vi "SMC_GetLimit.vi"(8 "error in (no error)":errorcluster) -> (0 "error out":errorcluster, 2 "MaxValues":dbl[](array[numeric]) format="%.6f", 3 "MinValues":dbl[](array[numeric]) format="%.6f")   [LabVIEW 2015]
uses:
  SMC_SubVIs.llb/SMC_ManagerMode.ctl
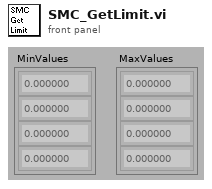
[diagram p1: front panel]
types:
  T1 = typedef "SMC_ManagerMode.ctl" = enum16{"Init", "Get", "SetPosition", "SetStatus", "SetMoving", "SetControllerNr"}
  T2 = typedef "SMC Paras.ctl" = cluster{"VENUS Language":T3, "Number of Axis":u8, "Controller Nr":u8, "Simulation":bool}
  T3 = typedef "VENUSNr.ctl" = enum16{"VENUS 2", "VENUS 1"}
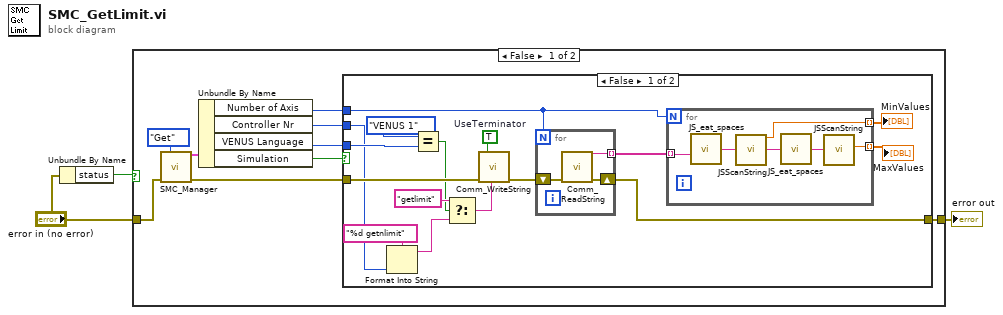
[diagram p0: block diagram]
diagram:
  n1 = Unbundle By Name("error in (no error)") -> ("status"=w3:bool)
  n2 = case shown="False" w3 {
    tunnel: "error in (no error)" -> [w11 w39]
    tunnel: [w9 w39] -> w1
    frame False {
      n3 = call "SMC_Manager.vi"("Mode"=SMC_ManagerMode."Get", "error in (no error)"=w11) -> ("SMC Parameter Out"=w8:T2, "error out"=w10:errorcluster)  [unwired: 9 in, 3 out]
      n4 = Unbundle By Name(w8) -> ("Number of Axis"=w5:u8, "Controller Nr"=w6:u8, "VENUS Language"=w7:T3, "Simulation"=w4:bool)
      n5 = case shown="False" w4 {
        tunnel: w10 -> [w25 w38]
        tunnel: [w23 w38] -> w9
        tunnel: w7 -> [w22 _]
        tunnel: w6 -> [w15 _]
        tunnel: w5 -> [w14 _]
        frame False {
          w13 = TRUE  # UseTerminator
          n6 = Format Into String(format string="%d getnlimit" ("Format String"), w15) -> (resulting string=w16:string)  [unwired: 2 in, 1 out]
          n7 = Equal?(x=enum16{"VENUS 2", "VENUS 1"}."VENUS 1", y=w22) -> (x = y?=w18:bool)
          n8 = Select(t="getlimit" ("Substring"), s=w18, f=w16) -> (s? t:f=w20:string)
          n9 = call "Comm_WriteString.vi"("string to write"=w20, "error in (no error)"=w25, "UseTerminator"=w13) -> ("error out"=w24:errorcluster)  [unwired: 8 in]
          n10 = for {
            N: w14 -> [_]
            shift-right: [w35] -> w23
            shift-left: w24 -> [w36]
            tunnel: [w37] -> w28 mode=indexing
            n11 = call "Comm_ReadString.vi"("error in (no error)"=w36) -> ("error out"=w35:errorcluster, "Answer"=w37:string)  [unwired: 9 in]
          }
          n12 = for {
            N: w14 -> [_]
            tunnel: [w31] -> w27 mode=indexing
            tunnel: w28 -> [w34] mode=indexing
            tunnel: [w30] -> w26 mode=indexing
            n13 = call "JS_eat_spaces.vi"("String In"=w34) -> ("String Out"=w33:string)
            n14 = call "JSScanString.vi"("String"=w33) -> ("result"=w31:dbl, "String Out"=w32:string)  [unwired: 9 in]
            n15 = call "JS_eat_spaces.vi"("String In"=w32) -> ("String Out"=w29:string)
            n16 = call "JSScanString.vi"("String"=w29) -> ("result"=w30:dbl)  [unwired: 9 in, 1 out]
          }
          "MinValues" <- w27
          "MaxValues" <- w26
        }
        frame True {
          # "Simulator"
        }
      }
    }
    frame True {
      # "Error, do nothing"
    }
  }
  "error out" <- w1
